vi "Stop_App.vi"(6 "Wash Entry":refnum<vi>, 8 "error in (no error)":errorcluster, 9 "Wash Options":refnum<vi>, 10 "This VI":refnum<vi>, 11 "Car Position":refnum<vi>) -> (0 "error out":errorcluster)   [LabVIEW 2023]
uses:
  9f675a26-981e-4937-a670-33123bfb0116.vi
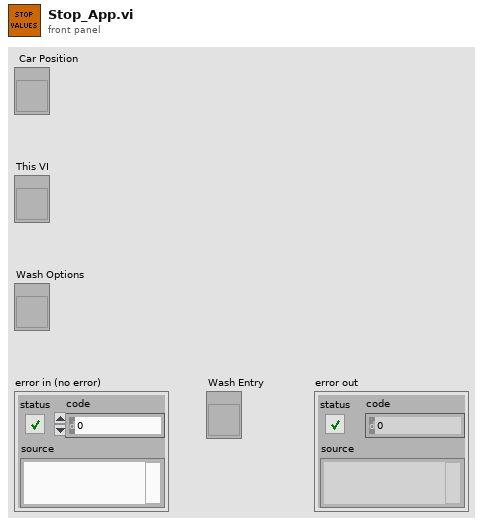
[diagram p1: front panel]
types:
  T1 = enum8{"Enabled", "Disabled", "Disabled and Grayed Out"}
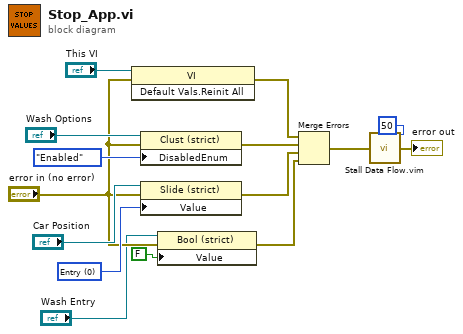
[diagram p0: block diagram]
diagram:
  w13 = u8 0 items=["Entry", "Station 1", "Station 2", "Station 3", "Exit"] ("Car Position Slider")
  n1 = invoke class="VI" method="Default Vals.Reinit All"(reference="This VI", error in="error in (no error)") -> (error out=w11:errorcluster)  [unwired: 1 in, 2 out]
  n2 = property class="Clust (strict)"(reference="Wash Options", error in="error in (no error)", "DisabledEnum"=T1."Enabled" ("Disabled")) -> (error out=w8:errorcluster)  [unwired: 1 out]
  n3 = property on="Property Node" class="Slide (strict)"(reference="Car Position", error in="error in (no error)", "Value"=w13) -> (error out=w7:errorcluster)  [unwired: 1 out]
  n4 = property class="Bool (strict)"(reference="Wash Entry", error in="error in (no error)", "Value"=FALSE) -> (error out=w5:errorcluster)  [unwired: 1 out]
  n5 = Merge Errors(w11, w8, w7, w5) -> (w9:errorcluster)
  n6 = call "Stall Data Flow.vim"("value in"=w9, "milliseconds to wait"=u32 50) -> ("value out"=→"error out":errorcluster)  [unwired: 1 out]
